vi "advertise.vi"(9 "type":string, 10 "topic":string) -> (3 "JSON string":string)   [LabVIEW 2014]
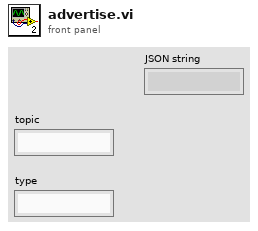
[diagram p1: front panel]
types:
  T1 = cluster{"op":string, "topic":string, "type":string}
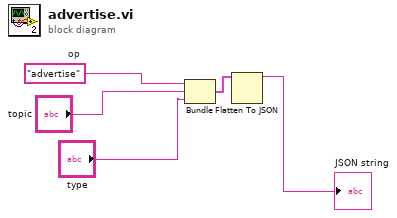
[diagram p0: block diagram]
diagram:
  w1 = "advertise"  # op
  n1 = Bundle("op"=w1, "topic"="topic", "type"="type") -> (w4:T1)  [unwired: 1 in]
  n2 = Flatten To JSON(anything=w4) -> (JSON string=→"JSON string":string)  [unwired: 2 in, 1 out]
